vi "Upd Flow Setpoint.vi"(8 "error in (no error)":errorcluster, 10 "Flow Setpoint":dbl, 11 "C100L in":refnum<class "C100L.lvclass">) -> (0 "error out":errorcluster, 3 "C100L out":refnum<class "C100L.lvclass">)   [LabVIEW 2021, in "C100L.lvlib" / "C100L.lvclass"]
uses:
  C100L.lvclass
  C100L.lvclass/C100L.ctl
  <vilib>/addons/control/pid/pid.llb/PID EGU to Percentage (DBL).vi
  <vilib>/addons/control/pid/pid.llb/PID Percentage to EGU (DBL).vi
  <vilib>/addons/control/pid/NI_PID_pid.lvlib
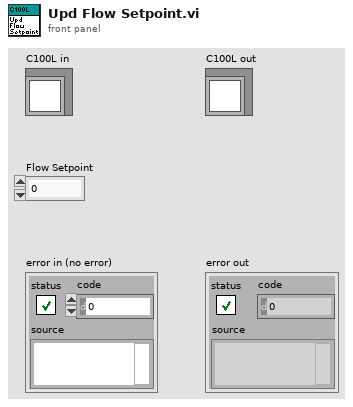
[diagram p1: front panel]
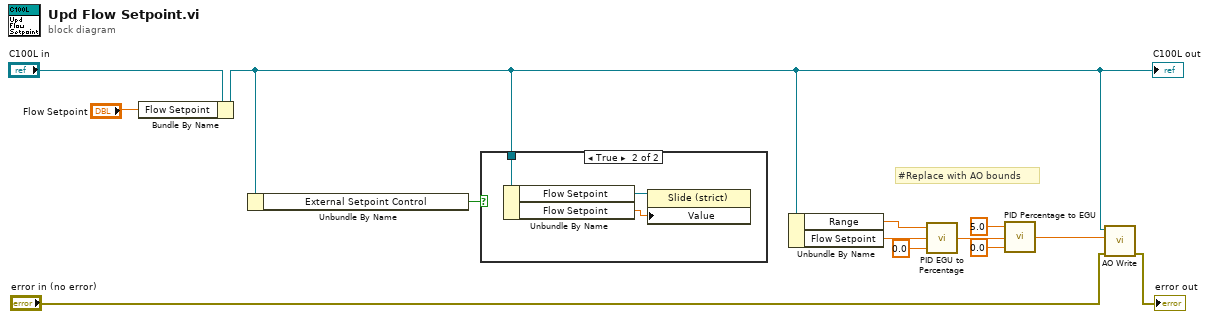
[diagram p0: block diagram]
diagram:
  # "#Replace with AO bounds"
  n1 = Bundle By Name(cluster="C100L in", "Flow Setpoint"="Flow Setpoint") -> (w3:refnum<class "C100L.lvclass">)
  "C100L out" <- w3
  n2 = Unbundle By Name(w3) -> ("External Setpoint Control"=w5:bool)
  n3 = case shown="True" w5 {
    tunnel: w3 -> [_ w16]
    frame False {
    }
    frame True {
      n4 = Unbundle By Name(w16) -> ("Flow Setpoint"=w15:refnum<vi>, "Flow Setpoint"=w14:dbl)
      n5 = property class="Slide (strict)"(reference=w15, "Value"=w14) -> ()  [unwired: 1 in, 2 out]
    }
  }
  n6 = Unbundle By Name(w3) -> ("Range"=w8:dbl, "Flow Setpoint"=w6:dbl)
  n7 = call-poly <vilib>:"PID EGU to Percentage.vi"("minimum (EGU)"=0.0, "input (EGU)"=w6, "maximum (EGU)"=w8) -> ("% span"=w9:dbl)
  n8 = call-poly <vilib>:"PID Percentage to EGU.vi"("minimum (EGU)"=0.0, "% span"=w9, "maximum (EGU)"=5.0) -> ("output (EGU)"=w4:dbl)  [unwired: 1 in]
  n9 = call "AO Write.vi"("error in (no error)"="error in (no error)", "Analog Output"=w4, "C100L in"=w3) -> ("error out"=→"error out":errorcluster)  [unwired: 8 in]
